vi "TDMS File Viewer.vi"(7 "file path":path) -> (0 "error out":errorcluster, 3 "file path out":path)   [LabVIEW 2014]
doc: "<B>Copyright:</B> (c) 2014 National Instruments. All rights reserved.\n\nOpens the .tdms file specified in the <B>file path</B> input and presents the file data in the TDMS File Viewer dialog box."
uses:
  <vilib>/Utility/tdmsutil.llb/fileViewerConfigData.ctl
  <vilib>/Utility/error.llb/DialogType.ctl
  <vilib>/event_ctls.llb/sizeaction.ctl
  <vilib>/event_ctls.llb/panelstate.ctl
  <vilib>/Utility/config.llb/Read Key (Path).vi
  <vilib>/Utility/tdmsutil.llb/TDMSFileViewerLocalizedText.vi
  Instance           1 26Saved   TDMS - File Viewer .vi
  <vilib>/Utility/config.llb/Write Key (Path).vi
  <vilib>/Utility/config.llb/NI_LVConfig.lvlib
  <vilib>/Utility/config.llb/Write Key (String).vi
panel:
  out "LastXScaleFormat":u8
  out "TotalCount":u64
  out "Temp Configuration":T1
  in  "LastTopLeftValue":u64
  out "Resize?":bool
  in  "Help":bool
  in  "Status":string
  in  "Quit":bool
  in  "Settings...":bool
  in  "Properties / Values / Graph":T2(tab)
  in  "Properties":i32(listbox)
  in  "Go To":bool
  in  "Scrollbar":u64(c297)
  in  "Raw data values":i32(listbox)
  out "Waveform Graph":waveform(dbl)[](graph)
  in  "File contents":string(tree)
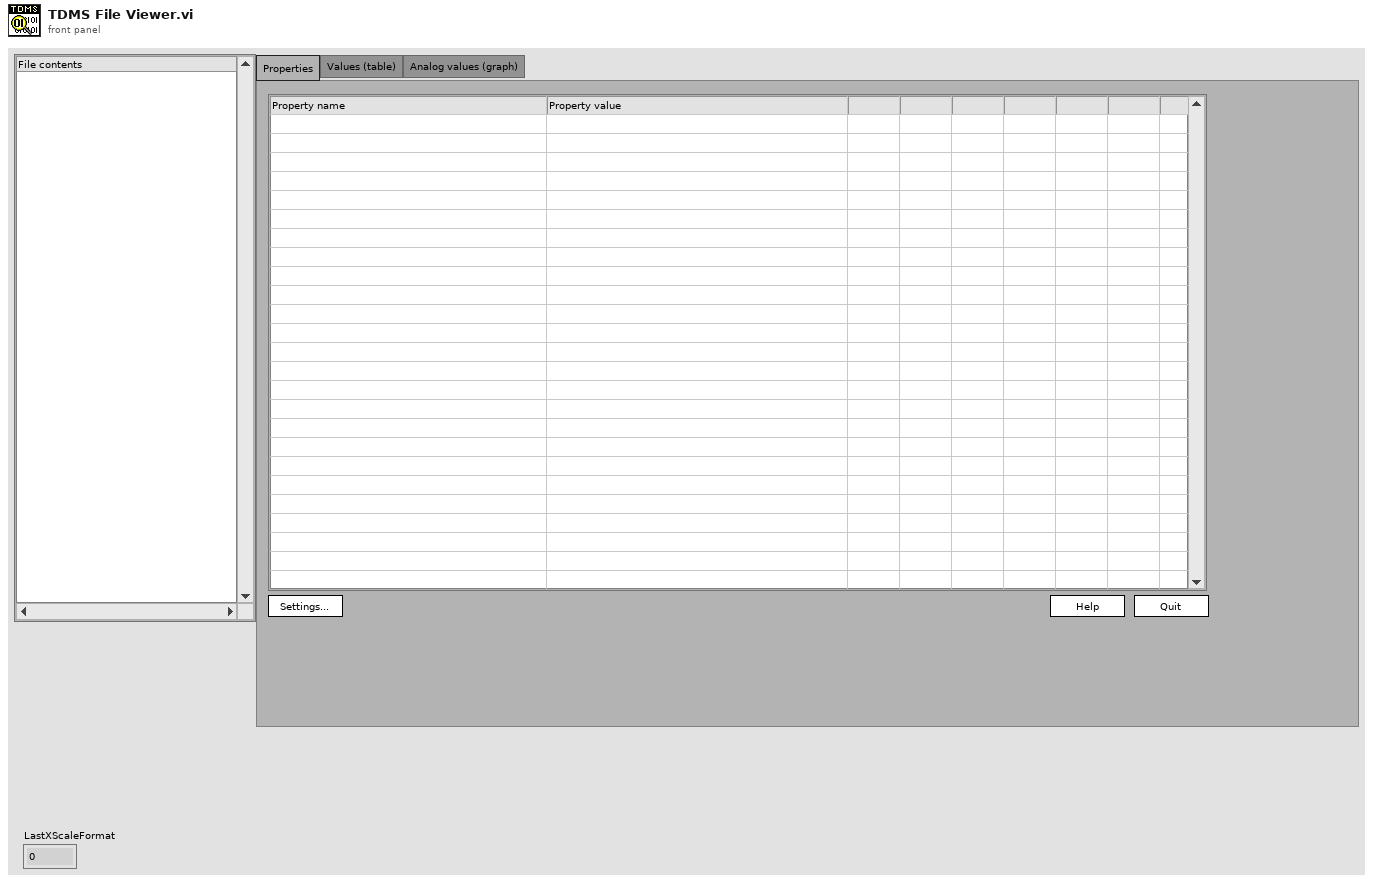
[diagram p1: front panel]
types:
  T1 = typedef "fileViewerConfigData.ctl" = cluster{"Show all (table)":bool, "Show all (graph)":bool, "limit (table)":u64, "limit (graph)":u64, "no show":bool, "start (table)":u64, "start (graph)":u64}
  T2 = enum32{"Properties", "Values (table)", "Analog values (graph)"}
  T3 = enum16{"open", "open or create", "create or replace", "create", "open (read-only)"}
  T4 = cluster{"Tree":refnum<vi>, "Tab Control":refnum<vi>, "property list":refnum<vi>, "raw data list":refnum<vi>, "Waveform Graph":refnum<vi>, "Ok":refnum<vi>, "Ok 2":refnum<vi>, "Ok 3":refnum<vi>, "Ok 4":refnum<vi>, "Scrollbar":refnum<vi>, "Ok 5":refnum<vi>, "TopLeftValue":refnum<vi>, "TotalCount":refnum<vi>}
  T5 = typedef "NI_LVConfig.lvlib/Config Data RefNum.ctl" = refnum<k1>
  T6 = typedef "panelstate.ctl" = enum32{"Standard", "Minimized", "Maximized"}
  T7 = typedef "sizeaction.ctl" = enum32{"Minimized", "Maximized", "Resized"}
  T8 = cluster{"Shift":bool, "Ctrl":bool, "Alt":bool, "Cmd":bool, "Opt":bool}
  T9 = typedef "LVRectTypeDef.ctl" = cluster{"Left":i16, "Top":i16, "Right":i16, "Bottom":i16}
  T10 = typedef "LVRowAndColumnUnsignedTypeDef.ctl" = cluster{"Row":u32, "Column":u32}
  T11 = typedef "DialogType.ctl" = u16
  T12 = typedef "eventvkey.ctl" = enum16{"ASCII", "Enter", "Return", "Shift", "Ctrl", "Alt", "Cmd", "Opt", "Caps", "NumLock", "Clear", "Break", "Up", "Down", "Left", "Right", "Insert", "Delete", "Home", "End", "PageUp", "PageDown", "Escape", "Help", "Pause", "ScrollLock", "F1", "F2", "F3", "F4", "F5", "F6", "F7", "F8", "F9", "F10", "F11", "F12", "F13", "F14", "F15", "F16", "F17", "F18", "F19", "F20", "F21", "F22", "F23", "F24", "Play", "VolumeUp", "VolumeDown", "Mute", "Two Byte Char"}
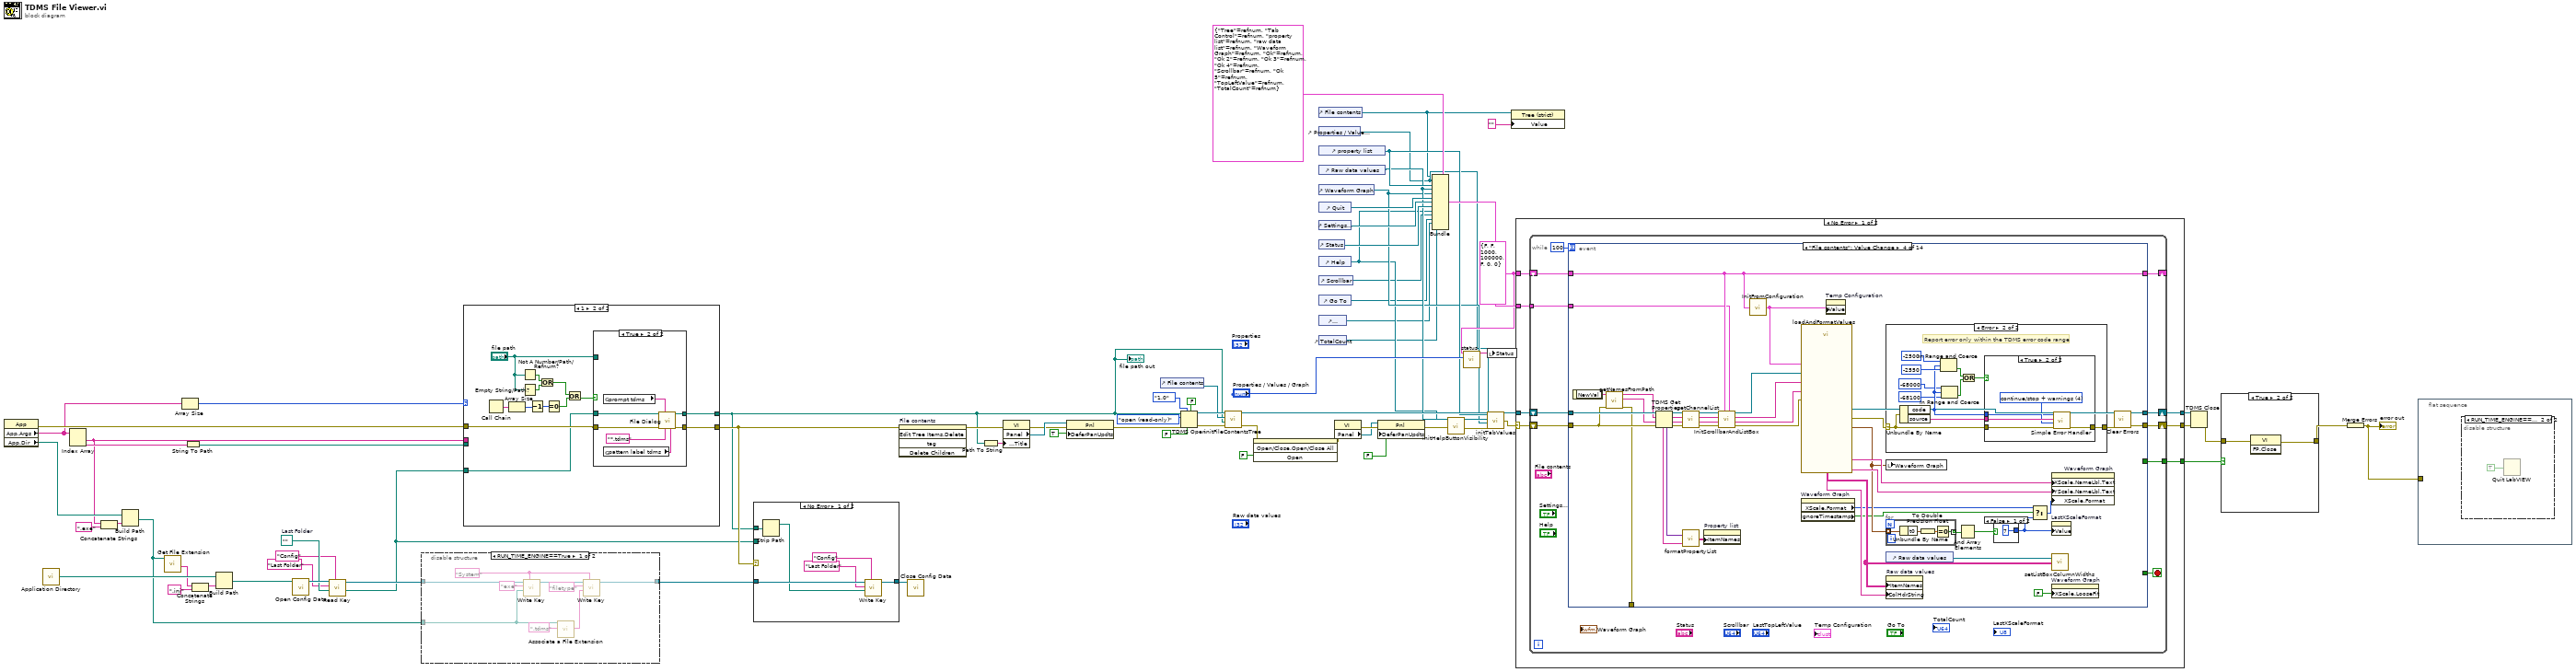
[diagram p0: block diagram]
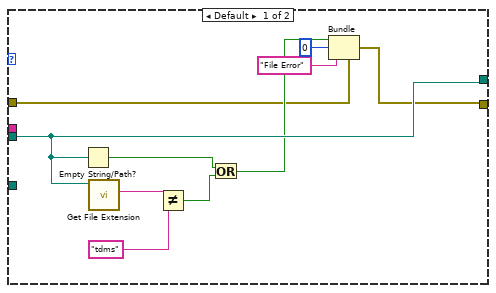
[diagram p4: hidden frame]
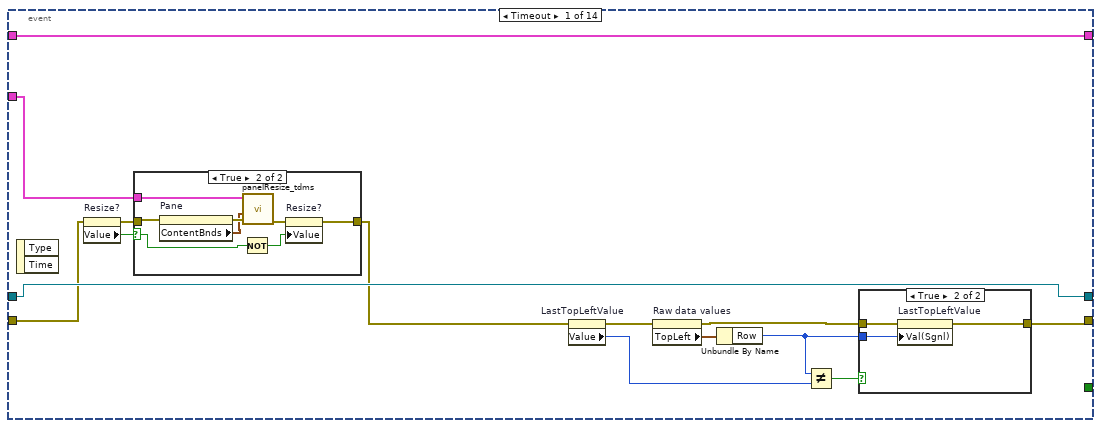
[diagram p8: hidden frame]
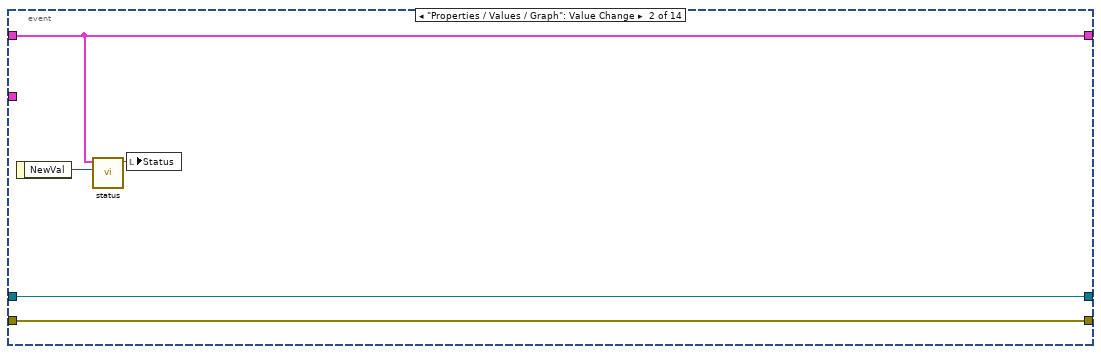
[diagram p11: hidden frame]
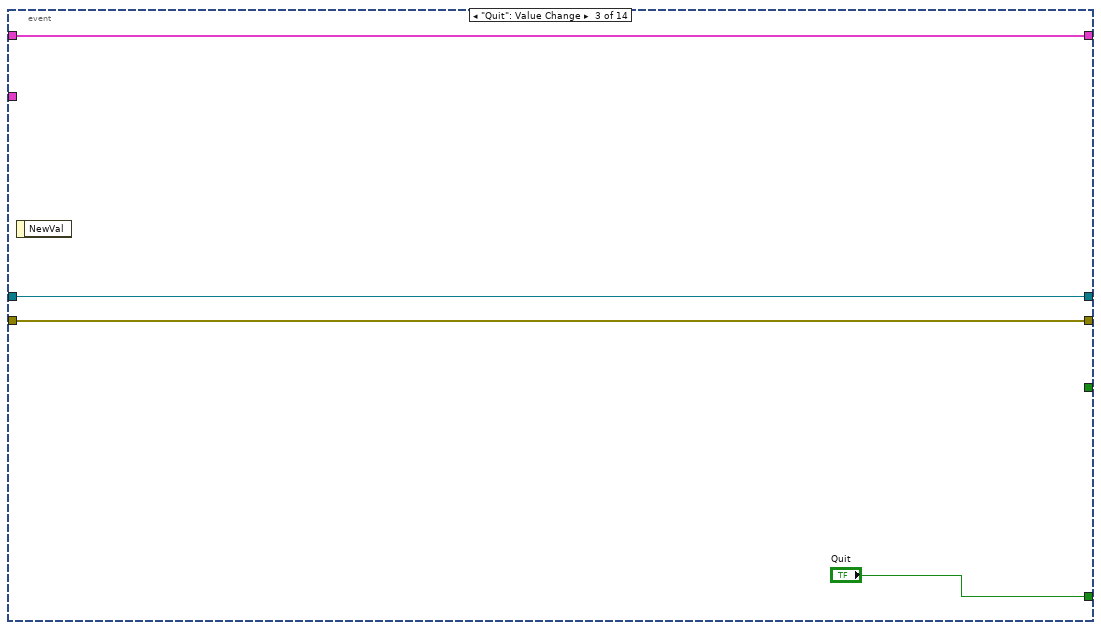
[diagram p12: hidden frame]
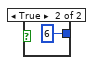
[diagram p13: hidden frame]
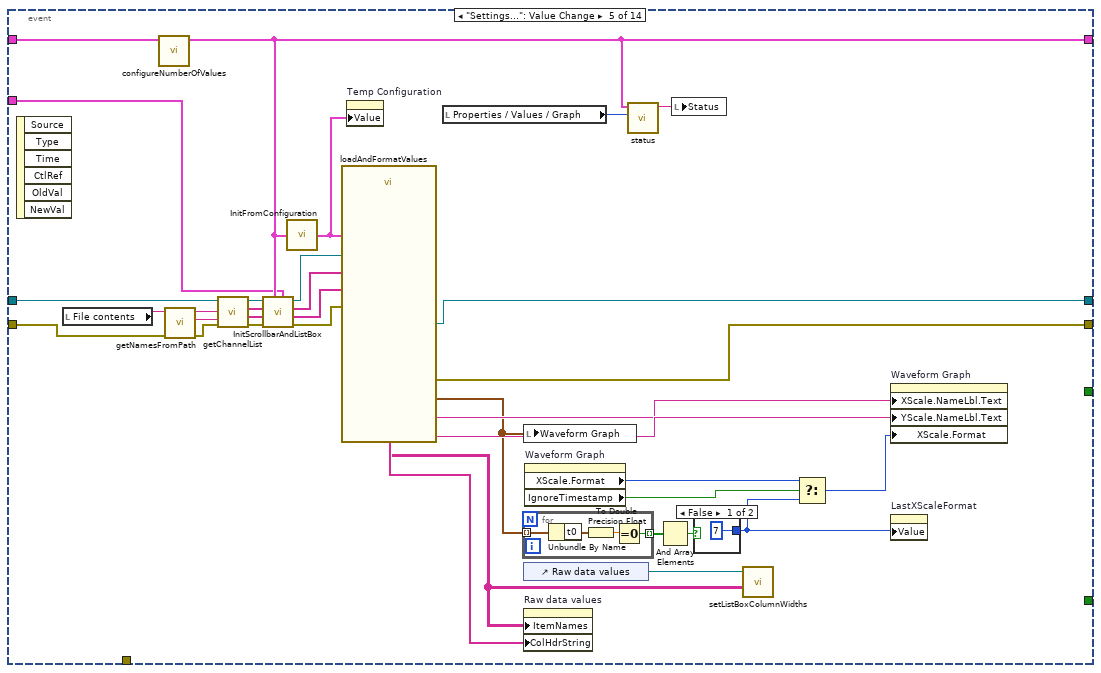
[diagram p16: hidden frame]
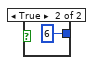
[diagram p17: hidden frame]
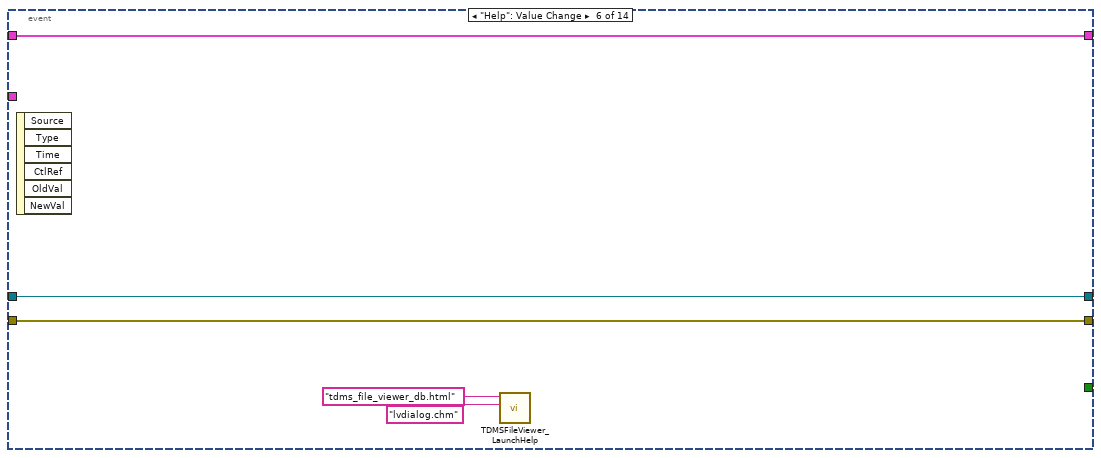
[diagram p18: hidden frame]
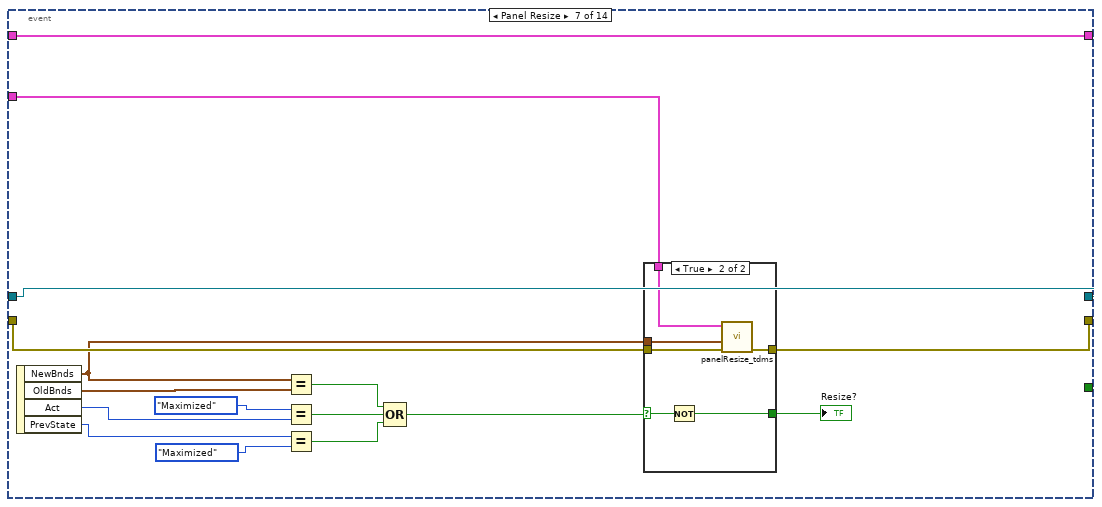
[diagram p19: hidden frame]
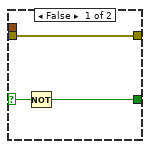
[diagram p20: hidden frame]
diagram:
  w4 = path ""  # Last Folder
  w49 = T1 {"Show all (table)"=FALSE, "Show all (graph)"=FALSE, "limit (table)"=1000, "limit (graph)"=100000, "no show"=FALSE, "start (table)"=0, "start (graph)"=0} ("TDMS File Viewer Configuration")
  n1 = property class="App"() -> (error out=w25:errorcluster, "App.Args"=w23:string[], "App.Dir"=w9:path)  [unwired: 2 in, 1 out]
  n2 = call <vilib>:"Application Directory.vi"() -> ("Application Directory"=w16:path)
  n3 = Index Array(array=w23) -> (element #1=w8:string, element #2=w24:string)  [unwired: 2 in]
  n4 = Concatenate Strings(w8, ".exe" ("string")) -> (w6:string)
  n5 = Build Path(base path=w9, name or relative path=w6) -> (appended path=w7:path)
  n6 = call <vilib>:"Get File Extension.vi"("file"=w7) -> ("filename without extension"=w13:string)  [unwired: 7 in, 3 out]
  n7 = Array Size(array=w23) -> (size(s)=w22:i32)
  n8 = String To Path(string=w24) -> (path=w21:path)
  n9 = Concatenate Strings(w13, ".ini" ("string")) -> (w17:string)
  n10 = Build Path(base path=w16, name or relative path=w17) -> (appended path=w12:path)
  n11 = call <vilib>:"Open Config Data.vi"("configuration file path"=w12) -> ("refnum"=w19:T5)  [unwired: 8 in, 2 out]
  n12 = call-poly <vilib>:"Read Key.vi"("section"="Config", "default value"=w4, "key"="Last Folder", "refnum"=w19) -> ("value"=w1:path, "refnum out"=w10:T5)  [unwired: 4 in, 2 out]
  n13 = disable-structure shown="RUN_TIME_ENGINE==True" {
    disable-tunnel: w7 -> [w74 _]
    disable-tunnel: [w78 w82] -> w11
    disable-tunnel: w10 -> [w81 w82]
    frame condition #0 {
      w77 = "System" ("section")
      w76 = ".tdms" ("string")
      n14 = call-poly <vilib>:"Write Key.vi"("section"=w77, "value"=w74, "key"="exe", "refnum"=w81) -> ("refnum out"=w79:T5)  [unwired: 5 in, 2 out]
      n15 = call "Associate a File Extension.vi"("string"=w76, "exe path"=w74) -> ()  [unwired: 8 in, 2 out]
      n16 = call-poly <vilib>:"Write Key.vi"("section"=w77, "value"=w76, "key"="filetype", "refnum"=w79) -> ("refnum out"=w78:T5)  [unwired: 5 in, 2 out]
    }
    frame condition #1 (active) {
    }
  }
  n17 = case shown="1" w22 {
    tunnel: [w84 w94] -> w15
    tunnel: [w92 w95] -> w14
    tunnel: w25 -> [w85 w96]
    tunnel: w21 -> [w92 _]
    tunnel: w8 -> [_ _]
    tunnel: w1 -> [_ w93]
    frame Default {
      n18 = Empty String/Path?(string/path=w92) -> (empty?=w89:bool)
      n19 = call <vilib>:"Get File Extension.vi"("file"=w92) -> ("lowercase file extension"=w91:string)  [unwired: 7 in, 3 out]
      n20 = Not Equal?(x=w91, y="tdms") -> (x != y?=w88:bool)
      n21 = Or(x=w89, y=w88) -> (x .or. y?=w87:bool)
      n22 = Bundle(cluster=w85, "status"=w87, "code"=0, "source"="File Error") -> (w84:errorcluster)
    }
    frame 1 {
      n23 = Call Chain() -> (call chain=w102:string[])
      n24 = Array Size(array=w102) -> (size(s)=w100:i32)
      n25 = Not A Number/Path/Refnum?(number/path/refnum="file path") -> (NaN/Path/Refnum?=w104:bool)
      n26 = Empty String/Path?(string/path="file path") -> (empty?=w103:bool)
      n27 = Decrement(x=w100) -> (x-1=w99:i32)
      n28 = Or(x=w104, y=w103) -> (x .or. y?=w101:bool)
      n29 = Equal To 0?(x=w99) -> (x = 0?=w97:bool)
      n30 = Or(x=w101, y=w97) -> (x .or. y?=w98:bool)
      n31 = case shown="True" w98 {
        tunnel: [w106 w113] -> w95
        tunnel: "file path" -> [w106 _]
        tunnel: [_ w111] -> w94
        tunnel: w96 -> [_ w108]
        tunnel: w93 -> [_ w107]
        frame False {
        }
        frame True {
          n32 = global read "TDMSFileViewerLocalizedText.vi" "prompt tdms"() -> (w110:string)
          n33 = global read "TDMSFileViewerLocalizedText.vi" "pattern label tdms"() -> (w109:string)
          n34 = call "File Dialog"("start path"=w107, "prompt"=w110, "error in"=w108, "pattern (all files)"="*.tdms", "pattern label"=w109) -> ("selected path"=w113:path, "error out"=w111:errorcluster)  [unwired: 2 in, 7 out]
        }
      }
    }
  }
  "file path out" <- w14
  n35 = case shown="No Error" w15 {
    tunnel: w11 -> [w119 w120]
    tunnel: w1 -> [_ _]
    tunnel: w14 -> [w118 _]
    tunnel: [w117 w120] -> w20
    frame No Error {
      n36 = Strip Path(path=w118) -> (stripped path=w116:path)  [unwired: 1 out]
      n37 = call-poly <vilib>:"Write Key.vi"("section"="Config", "value"=w116, "key"="Last Folder", "refnum"=w119) -> ("refnum out"=w117:T5)  [unwired: 5 in, 2 out]
    }
    frame Error {
    }
  }
  n38 = invoke on="File contents" class="Tree (strict)" method="Edit Tree Items.Delete"(error in=w15) -> (error out=w64:errorcluster)  [unwired: 4 in, 4 out]
  n39 = call <vilib>:"Close Config Data.vi"("refnum"=w20) -> ()  [unwired: 9 in, 2 out]
  n40 = Path To String(path=w14) -> (string=w26:string)
  n41 = property class="VI"(error in=w64, "Front Panel.Title"=w26) -> (error out=w65:errorcluster, "Panel"=w66:refnum<vi>)  [unwired: 1 in, 1 out]
  n42 = property class="Pnl"(reference=w66, error in=w65, "DeferPanUpdts"=TRUE ("Defer Panel Updates")) -> (error out=w68:errorcluster)  [unwired: 1 out]
  n43 = control-ref of="File contents"() -> (w52:refnum<vi>)
  n44 = TDMS Open(5:FALSE ("create index file? (T)"), 6:FALSE ("disable buffering (T)"), 7:enum16{"1.0", "2.0"}."1.0" ("file format version (2.0)"), 8:w68, 10:T3."open (read-only)" ("operation"), 11:w14) -> (0:w73:errorcluster, 3:w72:refnum<k34>)  [unwired: 1 in]
  n45 = call <vilib>:"initFileContentsTree.vi"("error in (no error)"=w73, "file path"=w14, "Tree Refnum"=w52, "tdms file"=w72) -> ("error out"=w60:errorcluster, "tdms file out"=w71:refnum<k34>)  [unwired: 2 out]
  n46 = invoke on="File contents" class="Tree (strict)" method="Open/Close.Open/Close All"(error in=w60, "Open"=FALSE ("Open?")) -> (error out=w59:errorcluster)  [unwired: 2 in, 3 out]
  n47 = control-ref of="File contents"() -> (w38:refnum<vi>)
  n48 = control-ref of="Properties / Values / Graph"() -> (w39:refnum<vi>)
  n49 = control-ref of="property list"() -> (w42:refnum<vi>)
  n50 = control-ref of="Raw data values"() -> (w41:refnum<vi>)
  n51 = control-ref of="Waveform Graph"() -> (w40:refnum<vi>)
  n52 = control-ref of="Quit"() -> (w56:refnum<vi>)
  n53 = control-ref of="Settings..."() -> (w54:refnum<vi>)
  n54 = control-ref of="Status"() -> (w51:refnum<vi>)
  n55 = control-ref of="Help"() -> (w34:refnum<vi>)
  n56 = control-ref of="Scrollbar"() -> (w32:refnum<vi>)
  n57 = control-ref of="Go To"() -> (w31:refnum<vi>)
  n58 = control-ref of="LastTopLeftValue"() -> (w30:refnum<vi>)
  n59 = control-ref of="TotalCount"() -> (w29:refnum<vi>)
  n60 = property class="VI"(error in=w59) -> (error out=w62:errorcluster, "Panel"=w61:refnum<vi>)  [unwired: 1 in, 1 out]
  n61 = property class="Pnl"(reference=w61, error in=w62, "DeferPanUpdts"=FALSE ("Defer Panel Updates")) -> (error out=w36:errorcluster)  [unwired: 1 out]
  n62 = Bundle(cluster=T4 {"Tree"=refnum, "Tab Control"=refnum, "property list"=refnum, "raw data list"=refnum, "Waveform Graph"=refnum, "Ok"=refnum, "Ok 2"=refnum, "Ok 3"=refnum, "Ok 4"=refnum, "Scrollbar"=refnum, "Ok 5"=refnum, "TopLeftValue"=refnum, "TotalCount"=refnum} ("control refs"), "Tree"=w38, "Tab Control"=w39, "property list"=w42, "raw data list"=w41, "Waveform Graph"=w40, "Ok"=w56, "Ok 2"=w54, "Ok 3"=w51, "Ok 4"=w34, "Scrollbar"=w32, "Ok 5"=w31, "TopLeftValue"=w30, "TotalCount"=w29) -> (w57:T4)
  n63 = call <vilib>:"initHelpButtonVisibility.vi"("error in"=w36, "Help"=w34) -> ("error out"=w35:errorcluster)  [unwired: 9 in]
  n64 = call <vilib>:"status.vi"("tab sheet"="Properties / Values / Graph", "TDMS File Viewer Configuration"=w49) -> ("status"=w50:string)  [unwired: 5 out]
  n65 = local write "Status"(w50) -> ()
  n66 = call <vilib>:"initTabValues.vi"("properties"=w42, "Values"=w41, "waveform"=w40, "error in"=w35, "Properties / Values / Graph"=w39) -> ("error out"=w43:errorcluster)
  n67 = property class="Tree (strict)"(reference=w38, "Value"="") -> ()  [unwired: 1 in, 2 out]
  n68 = case shown="No Error" w43 {
    selector: w43 -> [w122 w443]
    tunnel: w71 -> [w127 w444]
    tunnel: [w126 w444] -> w70
    tunnel: [w125 w443] -> w69
    tunnel: w57 -> [w124 _]
    tunnel: w49 -> [w123 _]
    tunnel: [w121 FALSE] -> w47
    frame No Error {
      n69 = while {
        shift-right: [w135] -> w125
        shift-left: w122 -> [w136]
        shift-right: [w134] -> w126
        shift-left: w127 -> [w137]
        tunnel: w124 -> [w132]
        shift-right: [w130] -> _
        shift-left: w123 -> [w131]
        tunnel: [w129] -> w121
        stop <- w133 stop-if-true
        n70 = event shown="[3] \"File contents\": Value Change" {
          selector: _ -> [_ _ _ _ _ _ _ _ _ _ _ _ _ _]
          dyn-events: _ -> [_ _ _ _ _ _ _ _ _ _ _ _ _ _]
          timeout: 100 -> [_ _ _ _ _ _ _ _ _ _ _ _ _ _]
          tunnel: w137 -> [w151 w168 w172 w214 w262 w282 w299 w310 w326 w345 w370 w385 w418 w435]
          tunnel: w136 -> [w146 w169 w171 w206 w269 w281 w297 _ w313 w337 w359 w382 w417 w434]
          tunnel: [w139 w169 w171 w202 w270 w281 w296 _ w320 w342 w362 w383 w417 w426] -> w135
          tunnel: [w151 w168 w172 w213 w271 w282 w299 w310 w325 w344 w369 w384 w418 w435] -> w134
          tunnel: [_ _ "Quit" _ _ _ _ w309 _ _ _ _ _ _] -> w133
          tunnel: [_ _ _ w205 _ _ _ _ _ _ _ _ _ _] -> _
          tunnel: w132 -> [w147 _ _ w181 w246 _ w298 _ w312 w338 w360 w379 _ _]
          tunnel: w131 -> [w150 w165 w170 w182 w272 w283 w295 _ w324 w346 w371 w386 w419 w436]
          tunnel: [w150 w165 w170 w182 w248 w283 w295 _ w324 w346 w371 w386 w419 w436] -> w130
          tunnel: [_ _ _ _ _ _ _ w309 _ _ _ _ _ _] -> w129
          event Timeout {
            n71 = event-data() -> ()  [unwired: 3 out]
            n72 = property on="Resize?" class="Bool (strict)"(error in=w146) -> (error out=w148:errorcluster, "Value"=w149:bool)  [unwired: 1 in, 1 out]
            n73 = case shown="True" w149 {
              selector: w149 -> [_ w163]
              tunnel: w147 -> [_ w164]
              tunnel: w148 -> [w156 w159]
              tunnel: [w156 w161] -> w144
              frame False {
              }
              frame True {
                n74 = property on="Pane" class="Pane"(error in=w159) -> (error out=w158:errorcluster, "ContentBnds"=w157:T9)  [unwired: 1 in, 1 out]
                n75 = Not(x=w163) -> (.not. x?=w160:bool)
                n76 = call <vilib>:"panelResize_tdms.vi"("error in (no error)"=w158, "NewBnds"=w157, "control refs"=w164) -> ("error out"=w162:errorcluster)  [unwired: 4 in]
                n77 = property on="Resize?" class="Bool (strict)"(error in=w162, "Value"=w160) -> (error out=w161:errorcluster)  [unwired: 1 in, 1 out]
              }
            }
            n78 = property on="LastTopLeftValue" class="DigNum (strict)"(error in=w144) -> (error out=w143:errorcluster, "Value"=w142:u64)  [unwired: 1 in, 1 out]
            n79 = property on="Raw data values" class="MCListbox (strict)"(error in=w143) -> (error out=w140:errorcluster, "TopLeft"=w145:T10)  [unwired: 1 in, 1 out]
            n80 = Unbundle By Name(w145) -> ("Row"=w138:u32)
            n81 = Not Equal?(x=w138, y=w142) -> (x != y?=w141:bool)
            n82 = case shown="True" w141 {
              tunnel: w140 -> [w152 w155]
              tunnel: [w152 w154] -> w139
              tunnel: w138 -> [_ w153]
              frame False {
              }
              frame True {
                n83 = property on="LastTopLeftValue" class="DigNum (strict)"(error in=w155, "Val(Sgnl)"=w153) -> (error out=w154:errorcluster)  [unwired: 1 in, 1 out]
              }
            }
          }
          event "Properties / Values / Graph": Value Change {
            n84 = event-data() -> ("NewVal"=w167:T2)  [unwired: 1 out]
            n85 = call <vilib>:"status.vi"("tab sheet"=w167, "TDMS File Viewer Configuration"=w165) -> ("status"=w166:string)  [unwired: 5 out]
            n86 = local write "Status"(w166) -> ()
          }
          event "Quit": Value Change {
            n87 = event-data() -> ()  [unwired: 2 out]
          }
          event "File contents": Value Change {
            n88 = event-data() -> ("NewVal"=w208:string)  [unwired: 1 out]
            n89 = call <vilib>:"getNamesFromPath.vi"("error in (no error)"=w206, "tree path"=w208) -> ("error out"=w205:errorcluster, "channel"=w211:string, "group"=w212:string)  [unwired: 3 out]
            n90 = TDMS Get Properties(8:w206, 9:w211, 10:w212, 11:w214) -> (0:w200:errorcluster, 1:w199:string, 2:w195:string, 3:w201:refnum<k34>, 4:w209:variant[], 6:w210:string[])  [unwired: 2 out]
            n91 = call <vilib>:"getChannelList.vi"("error in (no error)"=w200, "channel names"=w199, "group name"=w195, "tdms file"=w201) -> ("error out"=w190:errorcluster, "channel names out"=w188:string[], "group names out"=w186:string[], "tdms file out"=w184:refnum<k34>)
            n92 = call <vilib>:"formatPropertyList.vi"("property names"=w210, "property values"=w209) -> ("strings"=w207:string[][])
            n93 = property on="Property list" class="MCListbox (strict)"("ItemNames"=w207) -> ()  [unwired: 2 in, 2 out]
            n94 = call <vilib>:"InitScrollbarAndListBox.vi"("control refs"=w181, "configuration"=w182, "error in (no error)"=w190, "channel names"=w188, "group names"=w186, "tdms in"=w184) -> ("error out"=w189:errorcluster, "channel out"=w187:string[], "group out"=w185:string[], "tdms out"=w183:refnum<k34>)  [unwired: 2 in]
            n95 = call <vilib>:"InitFromConfiguration.vi"("configuration"=w182) -> ("output cluster"=w191:T1)  [unwired: 4 in]
            n96 = call <vilib>:"loadAndFormatValues.vi"("error in (no error)"=w189, "configuration"=w191, "channel names"=w187, "group names"=w185, "tdms file"=w183) -> ("error out"=w194:errorcluster, "graph y names"=w197:string, "graph x names"=w196:string, "tdms file out"=w213:refnum<k34>, "waveform values"=w180:waveform(dbl)[], "table values"=w204:string[][], "table headers"=w198:string[])
            n97 = property on="Waveform Graph" class="WFGraph (strict)"() -> ("XScale.Format"=w175:u8, "IgnoreTimestamp"=w174:bool)  [unwired: 2 in, 2 out]
            n98 = property on="Temp Configuration" class="Clust (strict)"("Value"=w191) -> ()  [unwired: 2 in, 2 out]
            n99 = case shown="Error" w194 {
              selector: w194 -> [w221 w231]
              tunnel: [w221 w230] -> w193
              frame No Error {
              }
              frame Error {
                # "Report error only within the TDMS error code range"
                n100 = Unbundle By Name(w231) -> ("code"=w227:i32, "source"=w232:string)
                n101 = In Range and Coerce(upper limit=-2500, x=w227, lower limit=-2550 ("upper limit")) -> (In Range?=w224:bool)  [unwired: 1 out]
                n102 = In Range and Coerce(upper limit=-68000, x=w227, lower limit=-68100) -> (In Range?=w223:bool)  [unwired: 1 out]
                n103 = Or(x=w224, y=w223) -> (x .or. y?=w222:bool)
                n104 = case shown="True" w222 {
                  tunnel: w232 -> [_ w238]
                  tunnel: w231 -> [w233 w237]
                  tunnel: [w233 w236] -> w230
                  tunnel: w227 -> [_ w234]
                  frame False {
                    # "Out of the range of TDMS\nerror code, we don't report\nthem."
                  }
                  frame True {
                    w235 = T11 4 items=["no dialog", "OK message", "continue or stop message", "OK message + warnings", "continue/stop + warnings"] ("type of dialog (OK msg:1)")
                    n105 = call <vilib>:"Simple Error Handler.vi"("error code (no error:0)"=w234, "error source (\" \")"=w238, "type of dialog (OK msg:1)"=w235, "error in (no error)"=w237) -> ("error out"=w236:errorcluster)  [unwired: 1 in, 4 out]
                  }
                }
              }
            }
            n106 = local write "Waveform Graph"(w180) -> ()
            n107 = for {
              tunnel: w180 -> [w220] mode=indexing
              tunnel: [w217] -> w179 mode=indexing
              n108 = Unbundle By Name(w220) -> ("t0"=w219:timestamp)
              n109 = To Double Precision Float(number=w219) -> (double precision float=w218:dbl)
              n110 = Equal To 0?(x=w218) -> (x = 0?=w217:bool)
            }
            n111 = control-ref of="Raw data values"() -> (w203:refnum<vi>)
            n112 = property on="Raw data values" class="MCListbox (strict)"("ItemNames"=w204, "ColHdrString"=w198) -> ()  [unwired: 2 in, 2 out]
            n113 = And Array Elements(Boolean array=w179) -> (logical AND=w178:bool)
            n114 = case shown="False" w178 {
              tunnel: [u8 7 u8 6] -> w176
              frame False {
              }
              frame True {
              }
            }
            n115 = Select(t=w175, s=w174, f=w176) -> (s? t:f=w177:u8)
            n116 = property on="Waveform Graph" class="WFGraph (strict)"("XScale.NameLbl.Text"=w196, "YScale.NameLbl.Text"=w197, "XScale.Format"=w177) -> ()  [unwired: 2 in, 2 out]
            n117 = property on="LastXScaleFormat" class="DigNum (strict)"("Value"=w176) -> ()  [unwired: 2 in, 2 out]
            n118 = call <vilib>:"setListBoxColumnWidths.vi"("table data"=w204, "MCListbox Refnum"=w203) -> ()  [unwired: 1 out]
            n119 = property on="Waveform Graph" class="WFGraph (strict)"("XScale.LooseFit"=FALSE ("X Scale.Loose Fit")) -> ()  [unwired: 2 in, 2 out]
            n120 = call <vilib>:"Clear Errors.vi"("error in (no error)"=w193) -> ("error out"=w202:errorcluster)  [unwired: 1 in, 5 out]
          }
          event "Settings...": Value Change {
            n121 = event-data() -> ()  [unwired: 7 out]
            n122 = local read "File contents"() -> (w263:string)
            n123 = call <vilib>:"configureNumberOfValues.vi"("TDMS File Viewer Configuration"=w272) -> ("TDMS File Viewer Configuration Out"=w248:T1)  [unwired: 10 out]
            n124 = call <vilib>:"getNamesFromPath.vi"("error in (no error)"=w269, "tree path"=w263) -> ("error out"=w261:errorcluster, "channel"=w259:string, "group"=w260:string)  [unwired: 3 out]
            n125 = call <vilib>:"getChannelList.vi"("error in (no error)"=w261, "channel names"=w259, "group name"=w260, "tdms file"=w262) -> ("error out"=w250:errorcluster, "channel names out"=w252:string[], "group names out"=w254:string[], "tdms file out"=w256:refnum<k34>)
            n126 = call <vilib>:"InitScrollbarAndListBox.vi"("control refs"=w246, "configuration"=w248, "error in (no error)"=w250, "channel names"=w252, "group names"=w254, "tdms in"=w256) -> ("error out"=w249:errorcluster, "channel out"=w251:string[], "group out"=w253:string[], "tdms out"=w255:refnum<k34>)  [unwired: 2 in]
            n127 = call <vilib>:"InitFromConfiguration.vi"("configuration"=w248) -> ("output cluster"=w247:T1)  [unwired: 4 in]
            n128 = call <vilib>:"loadAndFormatValues.vi"("error in (no error)"=w249, "configuration"=w247, "channel names"=w251, "group names"=w253, "tdms file"=w255) -> ("error out"=w270:errorcluster, "graph y names"=w265:string, "graph x names"=w264:string, "tdms file out"=w271:refnum<k34>, "waveform values"=w243:waveform(dbl)[], "table values"=w266:string[][], "table headers"=w268:string[])
            n129 = property on="Temp Configuration" class="Clust (strict)"("Value"=w247) -> ()  [unwired: 2 in, 2 out]
            n130 = local read "Properties / Values / Graph"() -> (w257:T2)
            n131 = for {
              tunnel: w243 -> [w278] mode=indexing
              tunnel: [w275] -> w245 mode=indexing
              n132 = Unbundle By Name(w278) -> ("t0"=w277:timestamp)
              n133 = To Double Precision Float(number=w277) -> (double precision float=w276:dbl)
              n134 = Equal To 0?(x=w276) -> (x = 0?=w275:bool)
            }
            n135 = local write "Waveform Graph"(w243) -> ()
            n136 = control-ref of="Raw data values"() -> (w267:refnum<vi>)
            n137 = property on="Raw data values" class="MCListbox (strict)"("ItemNames"=w266, "ColHdrString"=w268) -> ()  [unwired: 2 in, 2 out]
            n138 = property on="Waveform Graph" class="WFGraph (strict)"() -> ("XScale.Format"=w240:u8, "IgnoreTimestamp"=w239:bool)  [unwired: 2 in, 2 out]
            n139 = call <vilib>:"status.vi"("tab sheet"=w257, "TDMS File Viewer Configuration"=w248) -> ("status"=w258:string)  [unwired: 5 out]
            n140 = And Array Elements(Boolean array=w245) -> (logical AND=w244:bool)
            n141 = local write "Status"(w258) -> ()
            n142 = case shown="False" w244 {
              tunnel: [u8 7 u8 6] -> w241
              frame False {
              }
              frame True {
              }
            }
            n143 = call <vilib>:"setListBoxColumnWidths.vi"("table data"=w266, "MCListbox Refnum"=w267) -> ()  [unwired: 1 out]
            n144 = Select(t=w240, s=w239, f=w241) -> (s? t:f=w242:u8)
            n145 = property on="Waveform Graph" class="WFGraph (strict)"("XScale.NameLbl.Text"=w264, "YScale.NameLbl.Text"=w265, "XScale.Format"=w242) -> ()  [unwired: 2 in, 2 out]
            n146 = property on="LastXScaleFormat" class="DigNum (strict)"("Value"=w241) -> ()  [unwired: 2 in, 2 out]
          }
          event "Help": Value Change {
            n147 = event-data() -> ()  [unwired: 7 out]
            n148 = call <vilib>:"TDMSFileViewer_LaunchHelp.vi"("CHM or HLP filename (lvdialog.chm)"="lvdialog.chm", "HTML filename"="tdms_file_viewer_db.html") -> ()  [unwired: 1 in, 5 out]
          }
          event Panel Resize {
            n149 = event-data() -> ("NewBnds"=w287:T9, "OldBnds"=w286:T9, "Act"=w288:T7, "PrevState"=w289:T6)  [unwired: 1 out]
            n150 = Equal?(x=w287, y=w286) -> (x = y?=w292:bool)
            n151 = Equal?(x=sizeaction."Maximized" ("Act"), y=w288) -> (x = y?=w291:bool)
            n152 = Equal?(x=w289, y=panelstate."Maximized" ("PrevState")) -> (x = y?=w290:bool)
            n153 = Compound Arithmetic op=OR(w292, w291, w290) -> (w285:bool)
            n154 = case shown="True" w285 {
              selector: w285 -> [w301 w304]
              tunnel: w298 -> [_ w308]
              tunnel: w297 -> [w302 w307]
              tunnel: [w302 w306] -> w296
              tunnel: w287 -> [_ w305]
              tunnel: [w300 w303] -> w284
              frame False {
                n155 = Not(x=w301) -> (.not. x?=w300:bool)
              }
              frame True {
                n156 = Not(x=w304) -> (.not. x?=w303:bool)
                n157 = call <vilib>:"panelResize_tdms.vi"("error in (no error)"=w307, "NewBnds"=w305, "control refs"=w308) -> ("error out"=w306:errorcluster)  [unwired: 4 in]
              }
            }
            "Resize?" <- w284
          }
          event Panel Close? {
            w309 = TRUE
            n158 = event-data() -> ()  [unwired: 5 out]
            n159 = event-data("Discard?"=w309) -> ()  [unwired: 1 in, 1 out]
          }
          event "Scrollbar", "LastTopLeftValue": Value Change {
            n160 = event-data() -> ("CtlRef"=w318:refnum<vi>, "NewVal"=w315:u64, "OldVal"=w314:u64)  [unwired: 1 out]
            n161 = control-ref of="LastTopLeftValue"() -> (w317:refnum<vi>)
            n162 = Equal?(x=w317, y=w318) -> (x = y?=w316:bool)
            n163 = case shown="True" w316 {
              tunnel: w315 -> [_ w331]
              tunnel: w314 -> [_ w330]
              tunnel: w313 -> [w327 w329]
              tunnel: [w327 w328] -> w311
              frame False {
              }
              frame True {
                n164 = Subtract(x=w331, y=w330) -> (x-y=w333:u64)
                n165 = property on="Scrollbar" class="Scroll (strict)"(error in=w329) -> (error out=w335:errorcluster, "Value"=w334:u64)  [unwired: 1 in, 1 out]
                n166 = Add(x=w334, y=w333) -> (x+y=w332:u64)
                n167 = property on="Scrollbar" class="Scroll (strict)"(error in=w335, "Value"=w332) -> (error out=w328:errorcluster)  [unwired: 1 in, 1 out]
              }
            }
            n168 = property on="Temp Configuration" class="Clust (strict)"(error in=w311) -> (error out=w322:errorcluster, "Value"=w323:T1)  [unwired: 1 in, 1 out]
            n169 = call <vilib>:"UpdateBufferForMultiListBoxIfNecessary.vi"("control refs"=w312, "error in"=w322, "Buffer Configuration"=w323, "TDMS File Viewer Configuration"=w324, "tdms file in"=w326) -> ("error out"=w321:errorcluster, "BufferConfig out"=w319:T1, "tdms file out"=w325:refnum<k34>)  [unwired: 4 in]
            n170 = property on="Temp Configuration" class="Clust (strict)"(error in=w321, "Value"=w319) -> (error out=w320:errorcluster)  [unwired: 1 in, 1 out]
          }
          event "Raw data values": Key Down?; "Raw data values": event type 3.0.x8000000b {
            n171 = event-data() -> ("VKey"=w340:T12)  [unwired: 1 out]
            n172 = call <vilib>:"UpdateScrollbarBeforeKeyEvent.vi"("error in (no error)"=w337, "VKey"=w340, "control refs 2"=w338) -> ("error out"=w343:errorcluster, "LoadBuffer?"=w341:bool, "DiscardEvent?"=w339:bool)  [unwired: 6 in]
            n173 = case shown="True" w341 {
              tunnel: w346 -> [_ w354]
              tunnel: w345 -> [w347 w353]
              tunnel: [w347 w352] -> w344
              tunnel: w343 -> [w348 w349]
              tunnel: [w348 w351] -> w336
              tunnel: w338 -> [_ w350]
              frame False {
              }
              frame True {
                n174 = property on="Temp Configuration" class="Clust (strict)"(error in=w349) -> (error out=w357:errorcluster, "Value"=w358:T1)  [unwired: 1 in, 1 out]
                n175 = call <vilib>:"UpdateBufferForMultiListBoxIfNecessary.vi"("control refs"=w350, "error in"=w357, "Buffer Configuration"=w358, "TDMS File Viewer Configuration"=w354, "tdms file in"=w353) -> ("error out"=w356:errorcluster, "BufferConfig out"=w355:T1, "tdms file out"=w352:refnum<k34>)  [unwired: 4 in]
                n176 = property on="Temp Configuration" class="Clust (strict)"(error in=w356, "Value"=w355) -> (error out=w351:errorcluster)  [unwired: 1 in, 1 out]
              }
            }
            n177 = call <vilib>:"UpdateListBoxAfterKeyEvent.vi"("DiscardEvent?"=w339, "error in (no error)"=w336, "VKey"=w340, "control refs"=w338) -> ("error out"=w342:errorcluster)  [unwired: 7 in]
            n178 = event-data("Discard?"=w339) -> ()  [unwired: 1 in, 1 out]
          }
          event "Go To": Value Change {
            n179 = event-data() -> ()  [unwired: 2 out]
            n180 = call <vilib>:"GoTo.vi"("error in"=w359, "control refs"=w360) -> ("error out"=w368:errorcluster, "VisibleValue"=w365:u64)  [unwired: 8 in]
            n181 = property on="Temp Configuration" class="Clust (strict)"(error in=w368) -> (error out=w374:errorcluster, "Value"=w375:T1)  [unwired: 1 in, 1 out]
            n182 = call <vilib>:"UpdateBufferForMultiListBoxIfNecessary.vi"("control refs"=w360, "error in"=w374, "Buffer Configuration"=w375, "TDMS File Viewer Configuration"=w371, "tdms file in"=w370) -> ("error out"=w373:errorcluster, "BufferConfig out"=w372:T1, "tdms file out"=w369:refnum<k34>)  [unwired: 4 in]
            n183 = property on="Temp Configuration" class="Clust (strict)"(error in=w373, "Value"=w372) -> (error out=w361:errorcluster)  [unwired: 1 in, 1 out]
            n184 = property on="Raw data values" class="MCListbox (strict)"(error in=w361) -> (error out=w363:errorcluster, "TopLeft"=w367:T10)  [unwired: 1 in, 1 out]
            n185 = Unbundle By Name(w367) -> ("Row"=w366:u32)
            n186 = Add(x=w366, y=w365) -> (x+y=w364:u64)
            n187 = property on="Raw data values" class="MCListbox (strict)"(error in=w363, "Value"=w364) -> (error out=w362:errorcluster)  [unwired: 1 in, 1 out]
          }
          event Key Down {
            n188 = event-data() -> ("PlatMods"=w378:T8, "Char"=w377:i16)  [unwired: 1 out]
            n189 = property on="Raw data values" class="MCListbox (strict)"(error in=w382) -> (error out=w376:errorcluster, "Key Focus"=w381:bool)  [unwired: 1 in, 1 out]
            n190 = case shown="True" w381 {
              selector: w381 -> [w387 _]
              tunnel: [w387 w388] -> w380
              tunnel: w378 -> [_ w393]
              tunnel: w377 -> [_ w392]
              frame False {
              }
              frame True {
                n191 = disable-structure shown="Default" {
                  disable-tunnel: [T8 {"Shift"=FALSE, "Ctrl"=TRUE, "Alt"=FALSE, "Cmd"=FALSE, "Opt"=TRUE} ("PlatMods") T8 {"Shift"=FALSE, "Ctrl"=FALSE, "Alt"=FALSE, "Cmd"=TRUE, "Opt"=FALSE} ("PlatMods")] -> w394
                  frame condition #0 (active) {
                  }
                  frame condition #1 {
                  }
                }
                n192 = Equal?(x=w394, y=w393) -> (x = y?=w390:bool)
                n193 = Equal?(x=w392, y=i16 103 ("Char")) -> (x = y?=w389:bool)
                n194 = And(x=w390, y=w389) -> (x .and. y?=w388:bool)
              }
            }
            n195 = case shown="True" w380 {
              tunnel: w386 -> [_ w412]
              tunnel: w385 -> [w397 w411]
              tunnel: [w397 w410] -> w384
              tunnel: [w398 w403] -> w383
              tunnel: w376 -> [w398 w399]
              tunnel: w379 -> [_ w401]
              tunnel: w379 -> [_ w400]
              frame False {
              }
              frame True {
                n196 = call <vilib>:"GoTo.vi"("error in"=w399, "control refs"=w400) -> ("error out"=w409:errorcluster, "VisibleValue"=w406:u64)  [unwired: 8 in]
                n197 = property on="Temp Configuration" class="Clust (strict)"(error in=w409) -> (error out=w415:errorcluster, "Value"=w416:T1)  [unwired: 1 in, 1 out]
                n198 = call <vilib>:"UpdateBufferForMultiListBoxIfNecessary.vi"("control refs"=w401, "error in"=w415, "Buffer Configuration"=w416, "TDMS File Viewer Configuration"=w412, "tdms file in"=w411) -> ("error out"=w414:errorcluster, "BufferConfig out"=w413:T1, "tdms file out"=w410:refnum<k34>)  [unwired: 4 in]
                n199 = property on="Temp Configuration" class="Clust (strict)"(error in=w414, "Value"=w413) -> (error out=w402:errorcluster)  [unwired: 1 in, 1 out]
                n200 = property on="Raw data values" class="MCListbox (strict)"(error in=w402) -> (error out=w404:errorcluster, "TopLeft"=w408:T10)  [unwired: 1 in, 1 out]
                n201 = Unbundle By Name(w408) -> ("Row"=w407:u32)
                n202 = Add(x=w407, y=w406) -> (x+y=w405:u64)
                n203 = property on="Raw data values" class="MCListbox (strict)"(error in=w404, "Value"=w405) -> (error out=w403:errorcluster)  [unwired: 1 in, 1 out]
              }
            }
          }
          event Key Down? {
            n204 = event-data() -> ("VKey"=w421:T12)  [unwired: 1 out]
            n205 = case shown="\"F1\"" w421 {
              tunnel: [FALSE ("Discard?") TRUE ("Discard?")] -> w420
              frame Default {
              }
              frame "F1" {
                n206 = call <vilib>:"TDMSFileViewer_LaunchHelp.vi"("CHM or HLP filename (lvdialog.chm)"="lvdialog.chm", "HTML filename"="tdms_file_viewer_db.html") -> ()  [unwired: 1 in, 5 out]
              }
            }
            n207 = event-data("Discard?"=w420) -> ()  [unwired: 1 in, 1 out]
          }
          event "Waveform Graph": Shortcut Menu Selection (App) {
            n208 = event-data() -> ("ItemTag"=w432:string)  [unwired: 1 out]
            n209 = property on="Waveform Graph" class="WFGraph (strict)"(error in=w434) -> (error out=w427:errorcluster, "IgnoreTimestamp"=w431:bool)  [unwired: 1 in, 1 out]
            n210 = Not(x=w431) -> (.not. x?=w428:bool)
            n211 = Equal?(x=w432, y="APP_SC_IGNORE_TIME_STAMP") -> (x = y?=w429:bool)
            n212 = And(x=w428, y=w429) -> (x .and. y?=w430:bool)
            n213 = case shown="True" w430 {
              tunnel: w427 -> [w437 w441]
              tunnel: [w437 w438] -> w426
              frame False {
              }
              frame True {
                n214 = property on="LastXScaleFormat" class="DigNum (strict)"(error in=w441) -> (error out=w440:errorcluster, "Value"=w439:u8)  [unwired: 1 in, 1 out]
                n215 = property on="Waveform Graph" class="WFGraph (strict)"(error in=w440, "XScale.Format"=w439) -> (error out=w438:errorcluster)  [unwired: 1 in, 1 out]
              }
            }
          }
        }
      }
    }
    frame Error {
    }
  }
  n216 = TDMS Close(8:w69, 11:w70) -> (0:w46:errorcluster)  [unwired: 1 out]
  n217 = case shown="True" w47 {
    tunnel: w46 -> [w445 w447]
    tunnel: [w445 w446] -> w33
    frame False {
    }
    frame True {
      n218 = invoke class="VI" method="FP.Close"(error in=w447) -> (error out=w446:errorcluster)  [unwired: 2 in, 2 out]
    }
  }
  n219 = Merge Errors(w33) -> (w27:errorcluster)
  "error out" <- w27
  n220 = flat-sequence {
    tunnel: w27 -> [_]
    frame #0 {
      n221 = disable-structure shown="RUN_TIME_ENGINE==True" {
        frame condition #0 (active) {
        }
        frame condition #1 {
          n222 = Quit LabVIEW(quit? (T)=TRUE) -> ()
        }
      }
    }
  }
